vi "Filter Pairs.vi"(11 "Pairs":i64[](array[numeric])) -> (2 "Array 2":i32[](array[numeric]), 3 "Array":i64[](array[numeric]))   [LabVIEW 2020]
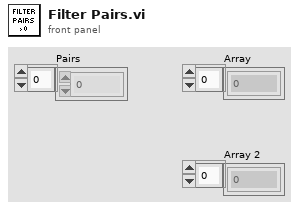
[diagram p1: front panel]
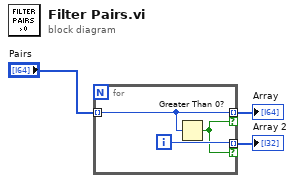
[diagram p0: block diagram]
diagram:
  n1 = for {
    tunnel: [w6] -> w1 mode=indexing if=w4
    tunnel: "Pairs" -> [w5] mode=indexing
    tunnel: [w5] -> w3 mode=indexing if=w4
    i -> [w6]
    n2 = Greater Than 0?(x=w5) -> (x > 0?=w4:bool)
  }
  "Array" <- w3
  "Array 2" <- w1
